vi "Omron TCP FINS-Example.vi"() -> ()   [LabVIEW 2016]
uses:
  Data Def/Omron TCP FINS-Connection Data.ctl
  Omron TCP FINS-Read Data(I16 Array).vi
  Omron TCP FINS-Read Data(I16 Element).vi
  Omron TCP FINS-Read Data(Boolean Element).vi
  Omron TCP FINS-Read Data(Boolean Array).vi
  Omron TCP FINS-Write Data(I16 Array).vi
  Omron TCP FINS-Write Data(I16 Element).vi
  Omron TCP FINS-Write Data(Boolean Element).vi
  Omron TCP FINS-Write Data(Boolean Array).vi
panel:
  out "Connect?":bool
  in  "Connect":bool
  in  "Connection Data":T1={"Server IP Address"="192.168.250.1", "Client IP Address"="192.168.250.44", "Port"=9600, "Timeout"=1000, "Unit Number"=0}
  out "Time":u32
  in  "Read Data":bool
  in  "Read Type":T2(tab)
  in  "Read Setting(I16 Array)":T3={"I/O Memory Address"=130, "Beginning Address"=0, "No. Of Items"=1} {"I/O Memory Address" items=["DM"=130, "CIO"=176, "WR"=177, "HR"=178, "AR"=179, "TIM"=137, "EM"=152]}
  out "Data(I16 Array)-Read":i16[](array[numeric])
  out "size(s)":i32
  in  "Read Setting(I16 Element)":T4={"I/O Memory Address"=130, "Data Address"=0} {"I/O Memory Address" items=["DM"=130, "CIO"=176, "WR"=177, "HR"=178, "AR"=179, "TIM"=137, "EM"=152]}
  out "Data(I16 Element)-Read":i16
  in  "Read Setting(Boolean Element)":T5={"I/O Memory Address"=130, "Data Address"=0, "Bit Index"=0} {"I/O Memory Address" items=["DM"=130, "CIO"=176, "WR"=177, "HR"=178, "AR"=179, "TIM"=137, "EM"=152]}
  out "Data(Boolean Element)-Read":bool
  in  "Read Setting(Boolean Array)":T4={"I/O Memory Address"=130, "Data Address"=0} {"I/O Memory Address" items=["DM"=130, "CIO"=176, "WR"=177, "HR"=178, "AR"=179, "TIM"=137, "EM"=152]}
  out "Data(Boolean Array)-Read":bool[](array[boolean])
  in  "Write Type":T2(tab)
  in  "Write Setting(I16 Array)":T6={"I/O Memory Address"=130, "Beginning Address"=0} {"I/O Memory Address" items=["DM"=130, "CIO"=176, "WR"=177, "HR"=178, "AR"=179, "TIM"=137, "EM"=152]}
  in  "Data(I16 Array)-Write":i16[](array[numeric])=[0]
  in  "Write Setting(I16 Element)":T4={"I/O Memory Address"=130, "Data Address"=0} {"I/O Memory Address" items=["DM"=130, "CIO"=176, "WR"=177, "HR"=178, "AR"=179, "TIM"=137, "EM"=152]}
  in  "Data(I16 Element)-Write":i16
  in  "Write Setting(Boolean Element)":T5={"I/O Memory Address"=130, "Data Address"=0, "Bit Index"=0} {"I/O Memory Address" items=["DM"=130, "CIO"=176, "WR"=177, "HR"=178, "AR"=179, "TIM"=137, "EM"=152]}
  in  "Data(Boolean Element)-Write":bool
  in  "Write Setting(Boolean Array)":T4={"I/O Memory Address"=130, "Data Address"=0} {"I/O Memory Address" items=["DM"=130, "CIO"=176, "WR"=177, "HR"=178, "AR"=179, "TIM"=137, "EM"=152]}
  in  "Data(Boolean Array)-Write":bool[](array[boolean])=[FALSE, FALSE, FALSE, FALSE, FALSE, FALSE, FALSE, FALSE, FALSE, FALSE, FALSE, FALSE, FALSE, FALSE, FALSE, FALSE]
  in  "Write Data":bool
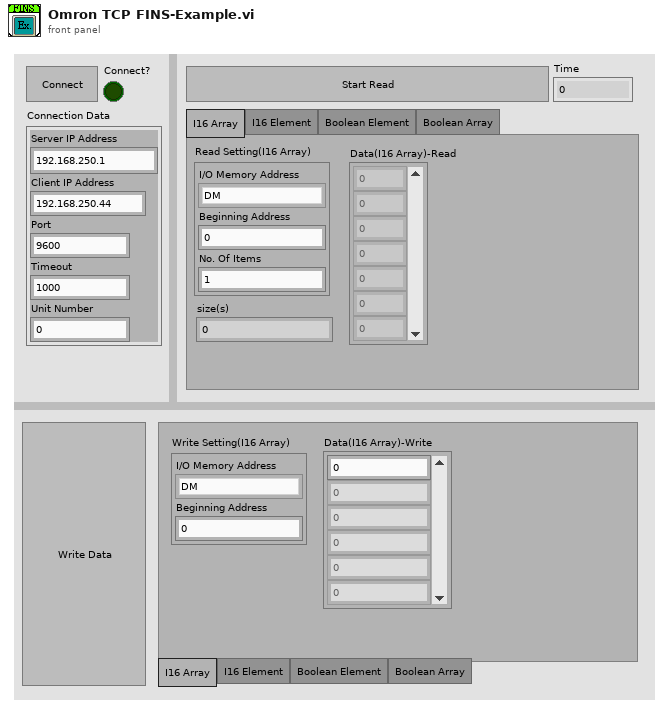
[diagram p1: front panel]
types:
  T1 = typedef "Omron TCP FINS-Connection Data.ctl" = cluster{"Server IP Address":string, "Client IP Address":string, "Port":u16, "Timeout":i32, "Unit Number":u8}
  T2 = enum32{"I16 Array", "I16 Element", "Boolean Element", "Boolean Array"}
  T3 = cluster{"I/O Memory Address":u8, "Beginning Address":u16, "No. Of Items":u16}
  T4 = cluster{"I/O Memory Address":u8, "Data Address":u16}
  T5 = cluster{"I/O Memory Address":u8, "Data Address":u16, "Bit Index":i32}
  T6 = cluster{"I/O Memory Address":u8, "Beginning Address":u16}
  T7 = typedef "Omron TCP FINS-Buffer Data.ctl" = cluster{"Connection ID":refnum<k5>, "Command Code":T8, "Command String":string, "Read Bytes":i32, "Response String":string, "Server Node":u8, "Client Node":u8, "Unit Number":u8}
  T8 = typedef "Omron TCP FINS-Command Code.ctl" = enum16{"Memory area read", "Memory area write"}
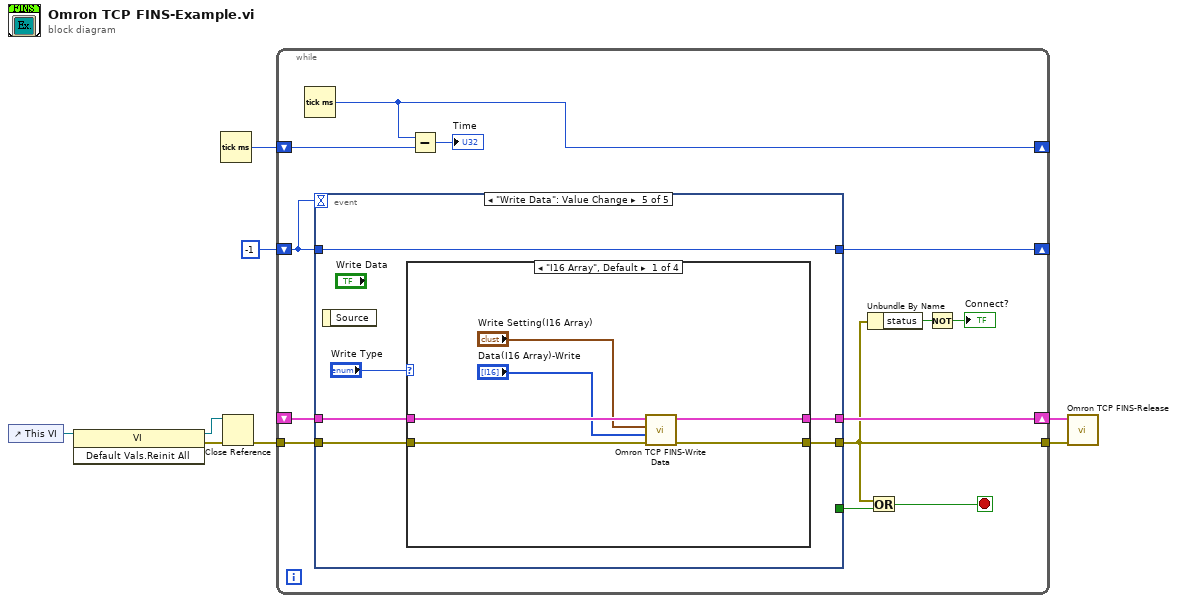
[diagram p0: block diagram]
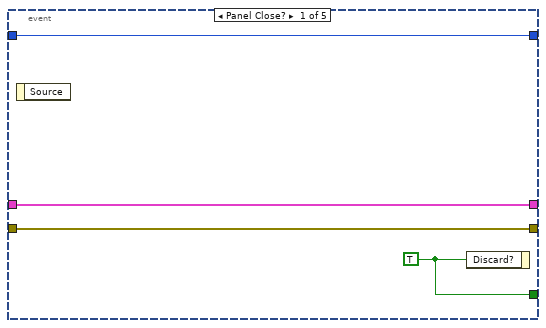
[diagram p2: hidden frame]
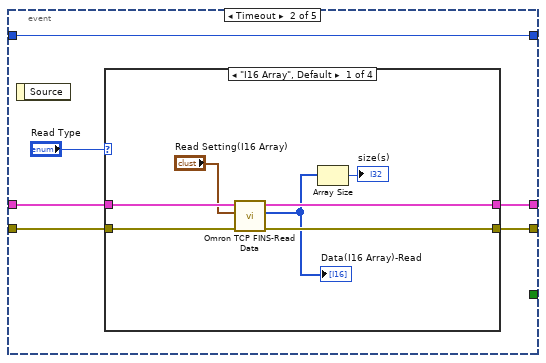
[diagram p3: hidden frame]
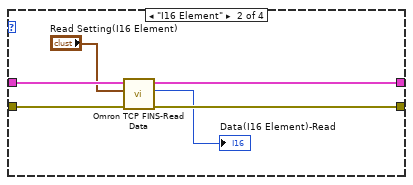
[diagram p4: hidden frame]
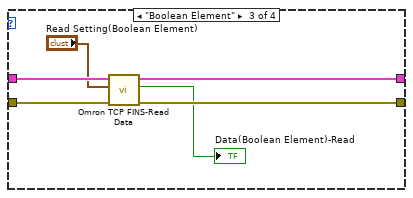
[diagram p5: hidden frame]
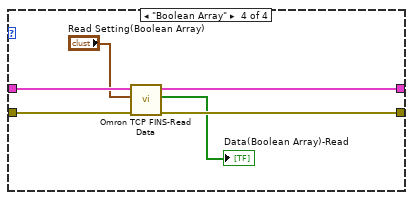
[diagram p6: hidden frame]
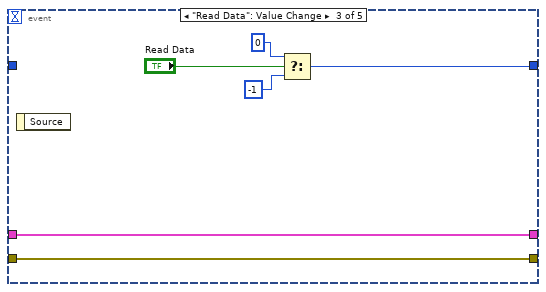
[diagram p7: hidden frame]
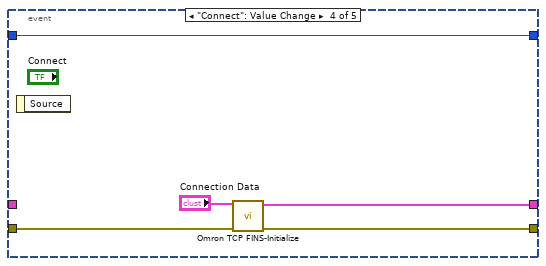
[diagram p8: hidden frame]
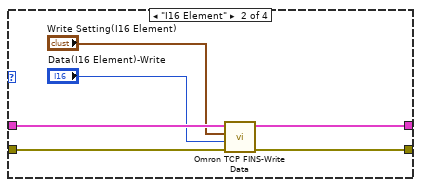
[diagram p9: hidden frame]
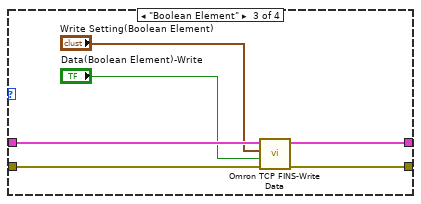
[diagram p10: hidden frame]
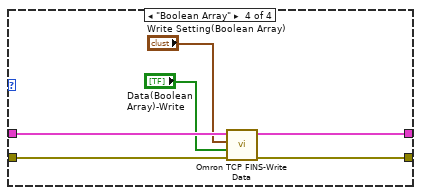
[diagram p11: hidden frame]
diagram:
  n1 = control-ref of="This VI"() -> (w5:refnum<vi>)
  n2 = invoke class="VI" method="Default Vals.Reinit All"(reference=w5) -> (reference out=w3:refnum<vi>, error out=w4:errorcluster)  [unwired: 2 in, 1 out]
  n3 = Tick Count (ms)() -> (millisecond timer value=w1:u32)
  n4 = Close Reference(reference=w3, error in (no error)=w4) -> (error out=w2:errorcluster)
  n5 = while {
    tunnel: w2 -> [w20]
    shift-right: [w17] -> w8
    shift-left: _ -> [w21]
    shift-right: [w18] -> _
    shift-left: -1 -> [w19]
    tunnel: [w14] -> w6
    shift-right: [w11] -> _
    shift-left: w1 -> [w10]
    stop <- w15 stop-if-true
    n6 = Tick Count (ms)() -> (millisecond timer value=w11:u32)
    n7 = event shown="[4] \"Write Data\": Value Change" {
      selector: _ -> [_ _ _ _ _]
      dyn-events: _ -> [_ _ _ _ _]
      timeout: w19 -> [_ _ _ _ _]
      tunnel: w21 -> [w24 w29 w61 _ w71]
      tunnel: w20 -> [w23 w28 w58 w65 w70]
      tunnel: w19 -> [w25 w31 _ w67 w73]
      tunnel: [w25 w31 w60 w67 w73] -> w18
      tunnel: [w24 w26 w61 w64 w69] -> w17
      tunnel: [w23 w27 w58 w63 w68] -> w14
      tunnel: [w22 _ _ _ _] -> w16
      event Panel Close? {
        w22 = TRUE ("Discard?")
        n8 = event-data() -> ()  [unwired: 1 in, 1 out]
        n9 = event-data("Discard?"=w22) -> ()  [unwired: 1 in, 1 out]
      }
      event Timeout {
        n10 = event-data() -> ()  [unwired: 1 in, 1 out]
        n11 = case shown="\"I16 Array\", Default" "Read Type" {
          tunnel: w29 -> [w38 w44 w50 w56]
          tunnel: w28 -> [w37 w43 w49 w55]
          tunnel: [w36 w42 w48 w54] -> w27
          tunnel: [w35 w41 w47 w53] -> w26
          frame "I16 Array", Default {
            n12 = call-poly "Omron TCP FINS-Read Data.vi"("error in"=w37, "Read Setting(I16 Array)"="Read Setting(I16 Array)", "Buffer Data In"=w38) -> ("error out"=w36:errorcluster, "Data"=w33:i16[], "Buffer Data Out"=w35:T7)  [unwired: 6 in]
            "Data(I16 Array)-Read" <- w33
            n13 = Array Size(array=w33) -> (size(s)=→"size(s)":i32)
          }
          frame "I16 Element" {
            n14 = call-poly "Omron TCP FINS-Read Data.vi"("error in"=w43, "Read Setting(I16 Element)"="Read Setting(I16 Element)", "Buffer Data In"=w44) -> ("error out"=w42:errorcluster, "Data"=→"Data(I16 Element)-Read":i16, "Buffer Data Out"=w41:T7)  [unwired: 6 in]
          }
          frame "Boolean Element" {
            n15 = call-poly "Omron TCP FINS-Read Data.vi"("error in"=w49, "Read Setting(Boolean Element)"="Read Setting(Boolean Element)", "Buffer Data In"=w50) -> ("error out"=w48:errorcluster, "Data"=→"Data(Boolean Element)-Read":bool, "Buffer Data Out"=w47:T7)  [unwired: 6 in]
          }
          frame "Boolean Array" {
            n16 = call-poly "Omron TCP FINS-Read Data.vi"("error in"=w55, "Read Setting(Boolean Array)"="Read Setting(Boolean Array)", "Buffer Data In"=w56) -> ("error out"=w54:errorcluster, "Data"=→"Data(Boolean Array)-Read":bool[], "Buffer Data Out"=w53:T7)  [unwired: 6 in]
          }
        }
      }
      event "Read Data": Value Change {
        n17 = event-data() -> ()  [unwired: 1 in, 1 out]
        n18 = Select(t=0, s="Read Data", f=-1) -> (s? t:f=w60:i32)
      }
      event "Connect": Value Change {
        n19 = event-data() -> ()  [unwired: 1 in, 1 out]
        n20 = call "Omron TCP FINS-Initialize.vi"("error in"=w65, "Connection Data In"="Connection Data") -> ("error out"=w63:errorcluster, "Buffer Data"=w64:T7)  [unwired: 8 in]
      }
      event "Write Data": Value Change {
        n21 = event-data() -> ()  [unwired: 1 in, 1 out]
        n22 = case shown="\"I16 Array\", Default" "Write Type" {
          tunnel: w71 -> [w79 w84 w91 w97]
          tunnel: w70 -> [w75 w85 w86 w96]
          tunnel: [w78 w83 w90 w95] -> w69
          tunnel: [w76 w82 w87 w94] -> w68
          frame "I16 Array", Default {
            n23 = call-poly "Omron TCP FINS-Write Data.vi"("error in"=w75, "Data"="Data(I16 Array)-Write", "Write Setting(I16 Array)"="Write Setting(I16 Array)", "Buffer Data In"=w79) -> ("error out"=w76:errorcluster, "Buffer Data Out"=w78:T7)  [unwired: 6 in]
          }
          frame "I16 Element" {
            n24 = call-poly "Omron TCP FINS-Write Data.vi"("error in"=w85, "Data"="Data(I16 Element)-Write", "Write Setting(I16 Element)"="Write Setting(I16 Element)", "Buffer Data In"=w84) -> ("error out"=w82:errorcluster, "Buffer Data Out"=w83:T7)  [unwired: 6 in]
          }
          frame "Boolean Element" {
            n25 = call-poly "Omron TCP FINS-Write Data.vi"("error in"=w86, "Data"="Data(Boolean Element)-Write", "Write Setting(Boolean Element)"="Write Setting(Boolean Element)", "Buffer Data In"=w91) -> ("error out"=w87:errorcluster, "Buffer Data Out"=w90:T7)  [unwired: 6 in]
          }
          frame "Boolean Array" {
            n26 = call-poly "Omron TCP FINS-Write Data.vi"("error in"=w96, "Data"="Data(Boolean Array)-Write", "Write Setting(Boolean Array)"="Write Setting(Boolean Array)", "Buffer Data In"=w97) -> ("error out"=w94:errorcluster, "Buffer Data Out"=w95:T7)  [unwired: 6 in]
          }
        }
      }
    }
    n27 = Subtract(x=w11, y=w10) -> (x-y=→"Time":u32)
    n28 = Unbundle By Name(w14) -> ("status"=w13:bool)
    n29 = Or(x=w14, y=w16) -> (x .or. y?=w15:bool)
    n30 = Not(x=w13) -> (.not. x?=→"Connect?":bool)
  }
  n31 = call "Omron TCP FINS-Release.vi"("error in"=w6, "Buffer Data"=w8) -> ()  [unwired: 9 in, 1 out]
